vi "ExampleGetSetJSON.vi"() -> ()   [LabVIEW 2019, in "LabJSON.lvlib"]
uses:
  LabJSON.lvlib
panel:
  in  "Numeric":dbl=123.76
  in  "Array - String":string[][](array[string])=[["Vegetables", "Count"], ["Carrot", "4"], ["Beetroot", "2"]]
  in  "Combo Box":string(combo)="Combo 1"
  in  "Enum":enum16{"One", "Two", "Three"}(ring)
  in  "File Path Control":path=path "C:/"
  in  "Table Control":string[][](table)=[["Fruits", "Count"], ["Apple", "10"], ["Orange", "12"]]
  in  "Command":T1(ring)
  out "JSON":string
  in  "Cluster":T2={"SubCluster"={"Array - Numeric"=[0.0, 1.2]}, "Numeric"=3.14, "Checkbox"=FALSE, "String"="Hello LabJSON!"}
  # "Example Usage:\n1. Choose command 'VI Controls to JSON'. Change values in below controls and run the VI.\n2. Change the values in JSON indicator, choose command 'JSON to VI Controls' and run the VI."
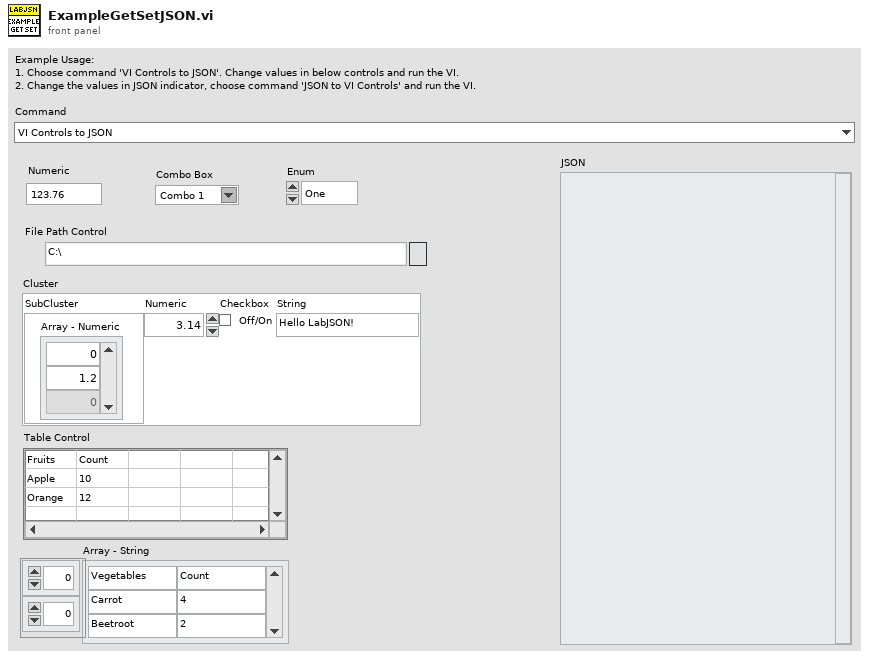
[diagram p1: front panel]
types:
  T1 = enum16{"VI Controls to JSON", "JSON to VI Controls"}
  T2 = cluster{"SubCluster":cluster{"Array - Numeric":dbl[]}, "Numeric":dbl, "Checkbox":bool, "String":string}
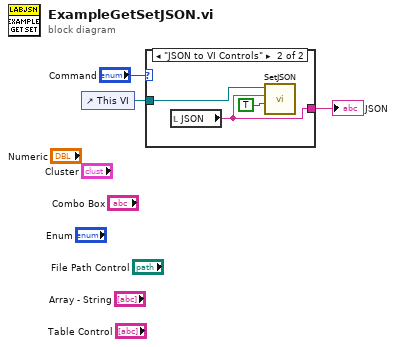
[diagram p0: block diagram]
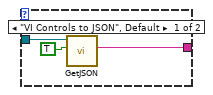
[diagram p2: hidden frame]
diagram:
  n1 = control-ref of="This VI"() -> (w3:refnum<vi>)
  n2 = case shown="\"JSON to VI Controls\"" "Command" {
    tunnel: w3 -> [w6 w9]
    tunnel: [w5 w8] -> w2
    frame "VI Controls to JSON", Default {
      n3 = call "GetJSON.vi"("Controls?"=TRUE, "VI Refnum In"=w6) -> ("JSON Out"=w5:string)  [unwired: 7 in, 2 out]
    }
    frame "JSON to VI Controls" {
      n4 = local read "JSON"() -> (w8:string)
      n5 = call "SetJSON.vi"("Controls?"=TRUE, "JSON Input"=w8, "VI Refnum In"=w9) -> ()  [unwired: 7 in, 2 out]
    }
  }
  "JSON" <- w2
